vi "Palette_Build Data.vi"(7 "Run Data":T1={"Target Folder"=path "", "Menu Folder"=path "", "Active Folder"=path "", "Config"={"Main"={"Menu Folder"="", "Re-Create Menu Folder?"=FALSE, "Allow mnu replace?"=FALSE}, "File Filter"={"Exclude Prefixes"=[], "Ignore Names"=[], "Include Extensions"=[], "Exclude Postfixes"=[]}, "Folder Filter"={"Exclude Prefixes"=[], "Ignore Names"=[]}, "File Name Edit"={"Pre Split String"="", "Post Split String"=""}, "Folder Name Edit"={"Pre Split String"="", "Post Split String"="", "Deletion Strings"=[]}, "Folder Icon Map"={}, "Default Palette Data"={"Display Name Override"="", "View Format"=2, "Palette Width"=0, "Help Tag"="", "Help File Path"=path "", "Palette Description"=""}, "Default File Data"={"Display Name Override"="", "Place VI Contents?"=FALSE}, "Palette Override map"={}, "File Override map"={}}} {"Config"."Default Palette Data"."View Format" items=["Icons", "Text", "Icons and Text"]}, 8 "error in (no error)":errorcluster, 11 "Element Array":T14[](array[typedef])) -> (0 "error out":errorcluster, 1 "Valid?":bool, 3 "palette data":T12 {"view format" items=["Icons", "Text", "Icons and Text"]})   [LabVIEW 2019, in "AutoMenuCreator.lvlib"]
uses:
  AutoMenuCreator.lvlib
  <vilib>/Palette API/Palette Menu/Public Type Define/Item.ctl
  <vilib>/Palette API/Palette Menu/Public Type Define/Palette Data.ctl
  <vilib>/Palette API/Palette Menu/Public Type Define/View Format.ctl
  <vilib>/Palette API/Palette Menu/Public Type Define/Items.ctl
  <vilib>/Palette API/Palette Menu/Public Type Define/Help Info.ctl
  <vilib>/Palette API/Palette Menu/Public Type Define/Synchronize Info.ctl
  Ctl/Ctl_Run Data.ctl
  Ctl/Ctl_Config.ctl
  Ctl/Ctl_Config_Main.ctl
  Ctl/Ctl_Config_File Filter.ctl
  Ctl/Ctl_Config_Folder Filter.ctl
  Ctl/Ctl_Config_File Name Edit.ctl
  Ctl/Ctl_Config_Folder Name Edit.ctl
  Ctl/Ctl_Config_Folder Icon Map.ctl
  Ctl/Ctl_Config_Palette Data.ctl
  <vilib>/Palette API/Palette Menu/Palette Menu.lvlib
  Ctl/Ctl_Config_File Data.ctl
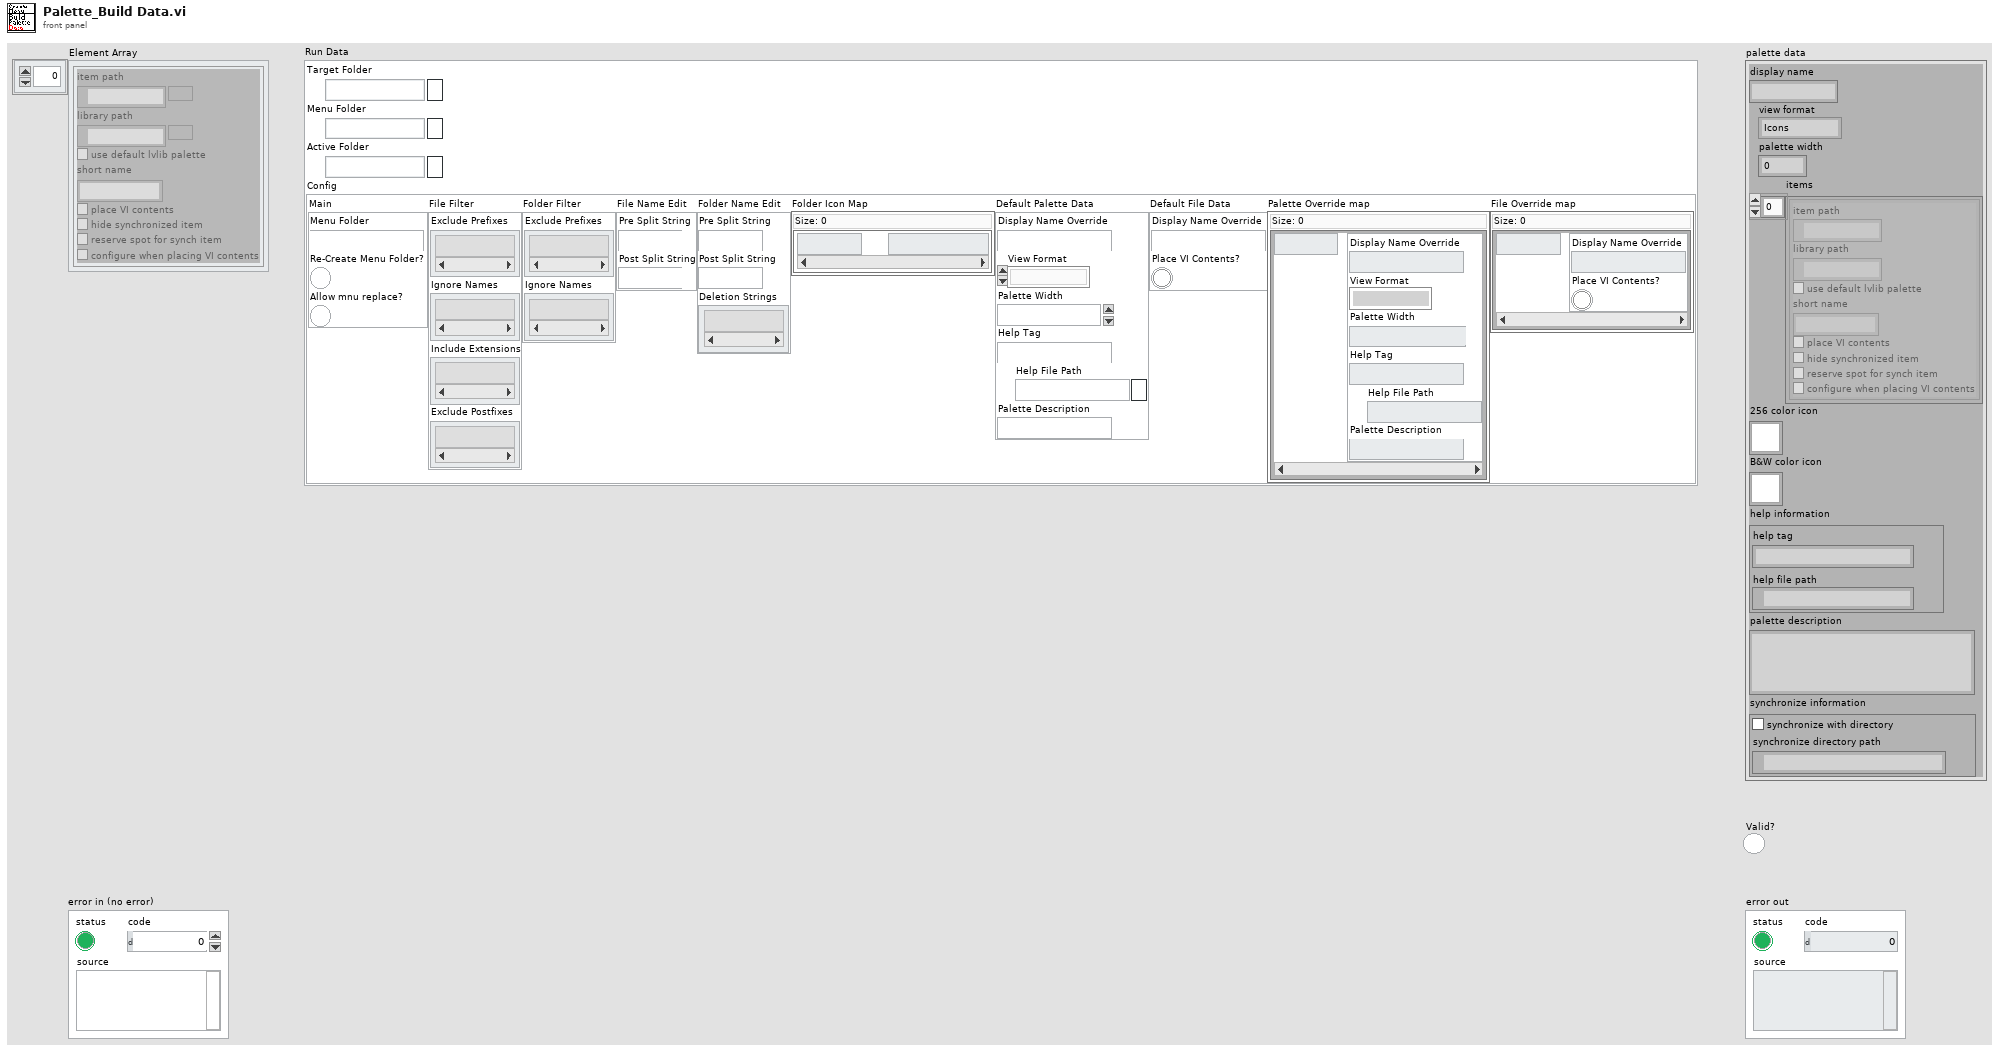
[diagram p1: front panel]
types:
  T1 = typedef "AutoMenuCreator.lvlib/Ctl_Run Data.ctl" = cluster{"Target Folder":path, "Menu Folder":path, "Active Folder":path, "Config":T2}
  T2 = typedef "AutoMenuCreator.lvlib/Ctl_Config.ctl" = cluster{"Main":T3, "File Filter":T4, "Folder Filter":T5, "File Name Edit":T6, "Folder Name Edit":T7, "Folder Icon Map":T8, "Default Palette Data":T9, "Default File Data":T11, "Palette Override map":map{string, T9}, "File Override map":map{string, T11}}
  T3 = typedef "AutoMenuCreator.lvlib/Ctl_Config_Main.ctl" = cluster{"Menu Folder":string, "Re-Create Menu Folder?":bool, "Allow mnu replace?":bool}
  T4 = typedef "AutoMenuCreator.lvlib/Ctl_Config_File Filter.ctl" = cluster{"Exclude Prefixes":string[], "Ignore Names":string[], "Include Extensions":string[], "Exclude Postfixes":string[]}
  T5 = typedef "AutoMenuCreator.lvlib/Ctl_Config_Folder Filter.ctl" = cluster{"Exclude Prefixes":string[], "Ignore Names":string[]}
  T6 = typedef "AutoMenuCreator.lvlib/Ctl_Config_File Name Edit.ctl" = cluster{"Pre Split String":string, "Post Split String":string}
  T7 = typedef "AutoMenuCreator.lvlib/Ctl_Config_Folder Name Edit.ctl" = cluster{"Pre Split String":string, "Post Split String":string, "Deletion Strings":string[]}
  T8 = typedef "AutoMenuCreator.lvlib/Ctl_Config_Folder Icon Map.ctl" = map{string, path}
  T9 = typedef "AutoMenuCreator.lvlib/Ctl_Config_Palette Data.ctl" = cluster{"Display Name Override":string, "View Format":T10, "Palette Width":i16, "Help Tag":string, "Help File Path":path, "Palette Description":string}
  T10 = typedef "Palette Menu.lvlib/View Format.ctl" = u16
  T11 = typedef "AutoMenuCreator.lvlib/Ctl_Config_File Data.ctl" = cluster{"Display Name Override":string, "Place VI Contents?":bool}
  T12 = typedef "Palette Menu.lvlib/Palette Data.ctl" = cluster{"display name":string, "view format":T10, "palette width":i16, "items":T13, "256 color icon":picture, "B&W color icon":picture, "help information":T15, "palette description":string, "synchronize information":T16}
  T13 = typedef "Palette Menu.lvlib/Items.ctl" = T14[]
  T14 = typedef "Palette Menu.lvlib/Item.ctl" = cluster{"item path":path, "library path":path, "use default lvlib palette":bool, "short name":string, "place VI contents":bool, "hide synchronized item":bool, "reserve spot for synch item":bool, "configure when placing VI contents":bool}
  T15 = typedef "Palette Menu.lvlib/Help Info.ctl" = cluster{"help tag":string, "help file path ":path}
  T16 = typedef "Palette Menu.lvlib/Synchronize Info.ctl" = cluster{"synchronize with directory":bool, "synchronize directory path":path}
  T17 = typedef "imagedata.ctl" = cluster{"image type":i32, "image depth":i32, "image":u8[], "mask":u8[], "colors":u32[], "Rectangle":cluster{"left":i16, "top":i16, "right":i16, "bottom":i16}}
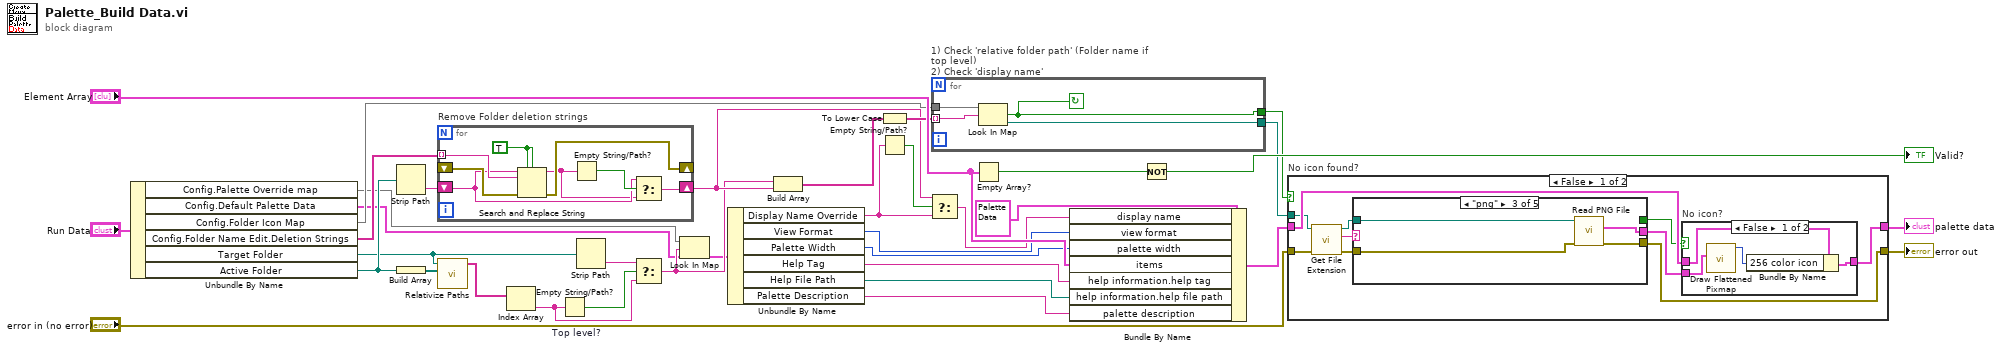
[diagram p0: block diagram]
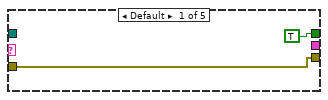
[diagram p3: hidden frame]
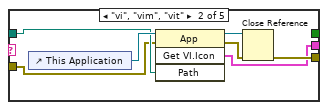
[diagram p4: hidden frame]
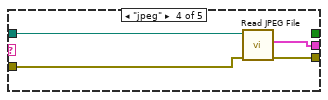
[diagram p5: hidden frame]
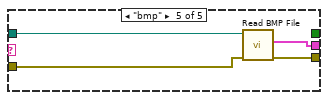
[diagram p6: hidden frame]
diagram:
  n1 = Unbundle By Name("Run Data") -> ("Config.Palette Override map"=w4:map{string, T9}, "Config.Default Palette Data"=w2:T9, "Config.Folder Icon Map"=w25:T8, "Config.Folder Name Edit.Deletion Strings"=w23:string[], "Target Folder"=w8:path, "Active Folder"=w22:path)
  n2 = Strip Path(path=w22) -> (name=w24:string)  [unwired: 1 out]
  n3 = Build Array(w22) -> (w21:path[])
  n4 = for "Remove Folder deletion strings" {
    shift-right: [w37] -> w15
    shift-left: w24 -> [w39]
    shift-right: [w44] -> _
    shift-left: _ -> [w43]
    tunnel: w23 -> [w42] mode=indexing
    w41 = TRUE ("ignore case? (F)")
    n5 = Search and Replace String(replace all?=w41, case sensitive?=w41, input string=w39, search string=w42, error in=w43) -> (result string=w38:string, error out=w44:errorcluster)  [unwired: 3 in, 2 out]
    n6 = Empty String/Path?(string/path=w38) -> (empty?=w40:bool)
    n7 = Select(t=w39, s=w40, f=w38) -> (s? t:f=w37:string)
  }
  n8 = call "Relativize Paths.vi"("Valid File Paths"=w21, "Target Folder"=w8) -> ("Array"=w20:string[])  [unwired: 9 in]
  n9 = Index Array(array=w20) -> (element=w5:string)  [unwired: 1 in]
  n10 = Empty String/Path? "Top level?"(string/path=w5) -> (empty?=w7:bool)
  n11 = Strip Path(path=w8) -> (name=w6:string)  [unwired: 1 out]
  n12 = Select(t=w6, s=w7, f=w5) -> (s? t:f=w3:string)
  n13 = Look In Map(map=w4, key=w3, default value=w2) -> (value=w1:T9)  [unwired: 1 out]
  n14 = Unbundle By Name(w1) -> ("Display Name Override"=w16:string, "View Format"=w13:T10, "Palette Width"=w12:i16, "Help Tag"=w11:string, "Help File Path"=w10:path, "Palette Description"=w9:string)
  n15 = Build Array(w3, w15) -> (w18:string[])
  n16 = To Lower Case(string=w18) -> (all lower case string=w27:string[])
  n17 = Empty String/Path?(string/path=w16) -> (empty?=w17:bool)
  n18 = Select(t=w15, s=w17, f=w16) -> (s? t:f=w14:string)
  n19 = for "1) Check 'relative folder path' (Folder name if top level)\n2) Check 'display name'" {
    tunnel: [w45] -> w32
    tunnel: [w48] -> w29
    tunnel: w27 -> [w47] mode=indexing
    tunnel: w25 -> [w46]
    stop <- w45 continue-if-true
    n20 = Look In Map(map=w46, key=w47) -> (key not found?=w45:bool, value=w48:path)  [unwired: 1 in]
  }
  n21 = Empty Array?(array="Element Array") -> (empty?=w35:bool)
  n22 = Bundle By Name(cluster=T12 {"display name"="", "view format"=2, "palette width"=4, "items"=[], "256 color icon"=bytes[0], "B&W color icon"=bytes[0], "help information"={"help tag"="", "help file path "=path ""}, "palette description"="", "synchronize information"={"synchronize with directory"=FALSE, "synchronize directory path"=path ""}} ("palette data"), "display name"=w14, "view format"=w13, "palette width"=w12, "items"="Element Array", "help information.help tag"=w11, "help information.help file path"=w10, "palette description"=w9) -> (w30:T12)
  n23 = Not(x=w35) -> (.not. x?=→"Valid?":bool)
  n24 = case "No icon found?" shown="False" w32 {
    tunnel: [w57 w86] -> w31
    tunnel: w30 -> [w58 w86]
    tunnel: w29 -> [w56 _]
    tunnel: [w52 w85] -> w28
    tunnel: "error in (no error)" -> [w50 w85]
    frame False {
      n25 = call <vilib>:"Get File Extension.vi"("error in (no error)"=w50, "file"=w56) -> ("error out"=w49:errorcluster, "lowercase file extension"=w55:string, "dup file"=w54:path)  [unwired: 5 in, 2 out]
      n26 = case shown="\"png\"" w55 {
        tunnel: w54 -> [_ w69 w76 w80 w84]
        tunnel: [TRUE _ _ _ _] -> w53
        tunnel: [w65 w67 w73 w78 w82] -> w52
        tunnel: w49 -> [w65 w68 w74 w79 w83]
        tunnel: [_ w66 w75 w77 w81] -> w51
        frame Default {
        }
        frame "vi", "vim", "vit" {
          n27 = control-ref of="This Application"() -> (w70:refnum<vi>)
          n28 = invoke class="App" method="Get VI.Icon"(reference=w70, error in=w68, "Path"=w69) -> (reference out=w71:refnum<vi>, error out=w72:errorcluster, "Get VI.Icon"=w66:T17)  [unwired: 1 in, 1 out]
          n29 = Close Reference(reference=w71, error in (no error)=w72) -> (error out=w67:errorcluster)
        }
        frame "png" {
          n30 = call <vilib>:"Read PNG File.vi"("error in (no error)"=w74, "path to PNG file"=w76) -> ("error out"=w73:errorcluster, "image data"=w75:T17)  [unwired: 7 in, 1 out]
        }
        frame "jpeg" {
          n31 = call <vilib>:"Read JPEG File.vi"("error in (no error)"=w79, "path to JPEG file"=w80) -> ("error out"=w78:errorcluster, "image data"=w77:T17)  [unwired: 7 in, 1 out]
        }
        frame "bmp" {
          n32 = call <vilib>:"Read BMP File.vi"("error in (no error)"=w83, "path to BMP file"=w84) -> ("error out"=w82:errorcluster, "image data"=w81:T17)  [unwired: 7 in, 1 out]
        }
      }
      n33 = case "No icon?" shown="False" w53 {
        tunnel: w58 -> [w62 w63]
        tunnel: [w61 w63] -> w57
        tunnel: w51 -> [w60 _]
        frame False {
          n34 = call <vilib>:"Draw Flattened Pixmap.vi"("image data"=w60) -> ("new picture"=w59:picture)  [unwired: 8 in]
          n35 = Bundle By Name(cluster=w62, "256 color icon"=w59) -> (w61:T12)
        }
        frame True {
        }
      }
    }
    frame True {
    }
  }
  "error out" <- w28
  "palette data" <- w31
